vi "test save binary file.vi"() -> ()   [LabVIEW 2018]
panel:
  out "Numeric":dbl
  out "error out":errorcluster
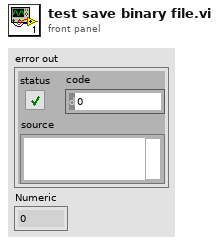
[diagram p1: front panel]
types:
  T1 = enum16{"big-endian, network order", "native, host order", "little-endian"}
  T2 = enum16{"open", "replace", "create", "open or create", "replace or create", "replace or create with confirmation"}
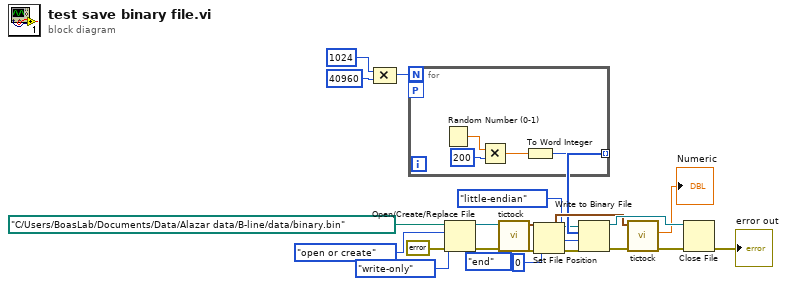
[diagram p0: block diagram]
diagram:
  n1 = Compound Arithmetic op=MULTIPLY(1024, 40960) -> (w22:i32)
  n2 = for {
    N: w22 -> [_]
    workers-P: _ -> [_]
    tunnel: [w23] -> w9 mode=indexing
    n3 = Random Number (0-1)() -> (number: 0 to 1=w26:dbl)
    n4 = Multiply(x=w26, y=200) -> (x*y=w24:dbl)
    n5 = To Word Integer(number=w24) -> (16bit integer=w23:i16)
  }
  n6 = Open/Create/Replace File(file path (use dialog)=path "C:/Users/BoasLab/Documents/Data/Alazar data/B-line/data/binary.bin", error in=errorcluster {"status"=FALSE, "code"=0, "source"=""}, operation (0:open)=T2."open or create", access (0:read/write)=enum16{"read/write", "read-only", "write-only"}."write-only") -> (refnum out=w6:refnum<file>, error out=w16:errorcluster)  [unwired: 2 in, 1 out]
  n7 = call "tictock.vi"("error in (no error)"=w16) -> ("error out"=w5:errorcluster, "seconds since 1Jan1904"=w11:timestamp)  [unwired: 8 in, 1 out]
  n8 = Set File Position(offset (in bytes) (0)=i64 0, refnum=w6, from (0:start)=enum16{"start", "end", "current"}."end", error in=w5) -> (refnum out=w3:refnum<file>, error out=w4:errorcluster)
  n9 = Write to Binary File(file (use dialog)=w3, data=w9, error in=w4, 9:T1."little-endian" ("byte order (0:big-endian, network order)")) -> (refnum out=w13:refnum<file>, error out=w15:errorcluster)  [unwired: 2 in, 1 out]
  n10 = call "tictock.vi"("error in (no error)"=w15, "seconds since 1Jan1904 2"=w11) -> ("error out"=w17:errorcluster, "Numeric"=→"Numeric":dbl)  [unwired: 7 in, 1 out]
  n11 = Close File(refnum=w13, error in=w17) -> (error out=→"error out":errorcluster)  [unwired: 1 out]
